vi "Type Panel.vi"(11 "ColumnPanel in":refnum<class "ColumnPanel.lvclass">) -> ()   [LabVIEW 2020, in "Conditum-Tools.lvlib" / "ColumnPanel.lvclass"]
uses:
  ColumnPanel.lvclass
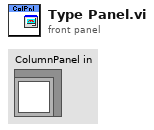
[diagram p1: front panel]
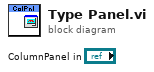
[diagram p0: block diagram]
diagram:
